vi "set_shutter.vi"(8 "error in (no error)":errorcluster, 10 "shutter open?":bool=TRUE, 11 "LightSourceMH110125Tsunami in":refnum<class "LightSourceMH110125Tsunami.lvclass">) -> (0 "error out":errorcluster, 2 "shutter open out?":bool, 3 "LightSourceMH110125Tsunami out":refnum<class "LightSourceMH110125Tsunami.lvclass">)   [LabVIEW 2010, in "LightSourceMH110125Tsunami.lvclass"]
uses:
  LightSourceMH110125Tsunami.lvclass
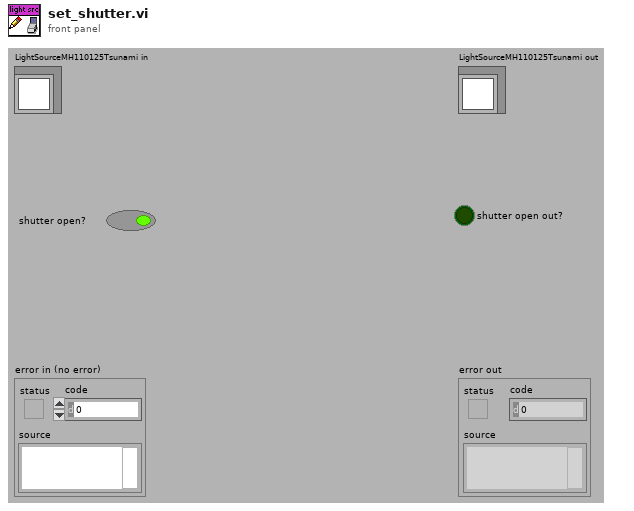
[diagram p1: front panel]
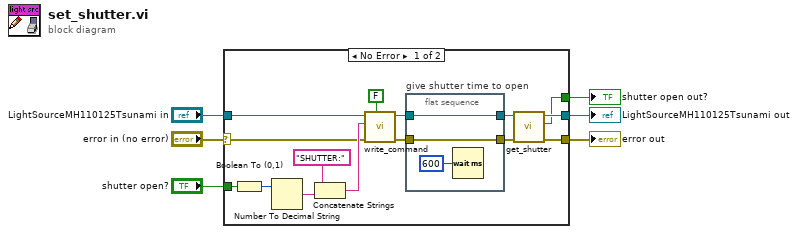
[diagram p0: block diagram]
diagram:
  n1 = case shown="No Error" "error in (no error)" {
    selector: "error in (no error)" -> [w7 w26]
    tunnel: [w16 w26] -> w1
    tunnel: [w15 w25] -> w3
    tunnel: "LightSourceMH110125Tsunami in" -> [w8 w25]
    tunnel: "shutter open?" -> [w21 _]
    tunnel: [w13 _] -> w2
    frame No Error {
      n2 = Boolean To (0,1)(Boolean=w21) -> (0, 1=w20:i16)
      n3 = Number To Decimal String(number=w20) -> (decimal integer string=w19:string)  [unwired: 1 in]
      n4 = Concatenate Strings("SHUTTER:", w19) -> (w17:string)
      n5 = call-dynamic "write_command.vi"("error in (no error)"=w7, "read (T)"=FALSE, "string to write"=w17, "LightSourceMH110125Tsunami in"=w8) -> ("error out"=w11:errorcluster, "LightSourceMH110125Tsunami out"=w12:refnum<class "LightSourceMH110125Tsunami.lvclass">)  [unwired: 5 in, 1 out]
      n6 = flat-sequence "give shutter time to open" {
        tunnel: w12 -> [w23]
        tunnel: w11 -> [w24]
        tunnel: [w24] -> w10
        tunnel: [w23] -> w9
        frame #0 {
          n7 = Wait (ms)(milliseconds to wait=u32 600) -> ()  [unwired: 1 out]
        }
      }
      n8 = call-dynamic "get_shutter.vi"("error in (no error)"=w10, "LightSourceMH110125Tsunami in"=w9) -> ("error out"=w16:errorcluster, "shutter open out?"=w13:bool, "LightSourceMH110125Tsunami out"=w15:refnum<class "LightSourceMH110125Tsunami.lvclass">)  [unwired: 7 in]
    }
    frame Error {
    }
  }
  "error out" <- w1
  "LightSourceMH110125Tsunami out" <- w3
  "shutter open out?" <- w2
